vi "Jumps_Globals.vi"() -> ()   [LabVIEW 2021]
panel:
  in  "Jumps 6":dbl[][](array[numeric])
  in  "Jumps 5":dbl[][](array[numeric])
  in  "Jumps 4":dbl[][](array[numeric])
  in  "Jumps 3":dbl[][](array[numeric])
  in  "Jumps 2":dbl[][](array[numeric])
  in  "Jumps":dbl[][](array[numeric])
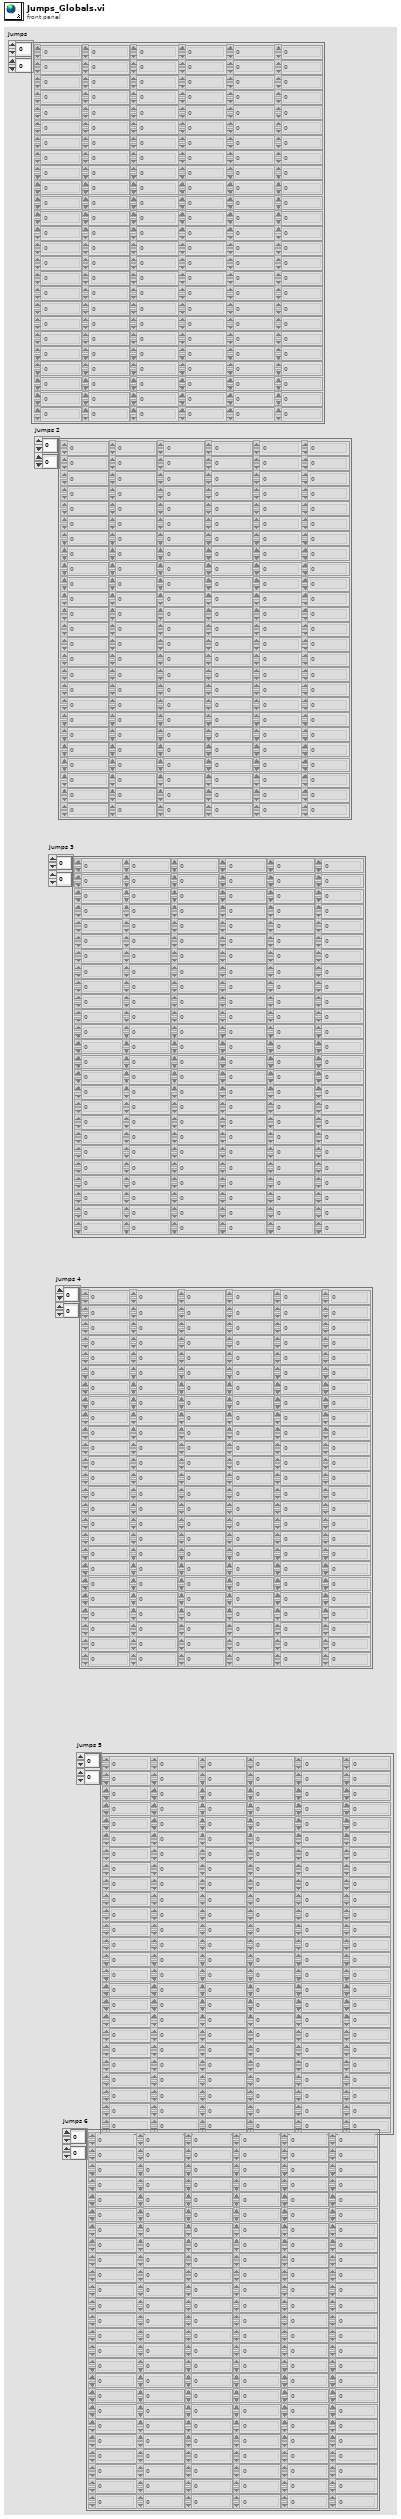
[diagram p1: front panel]
diagram:
